vi "WPILib Camera Set Attributes From File.vi"(8 "error in":errorcluster, 10 "Config Path":path, 11 "CameraDevRef":T1) -> (0 "error out":errorcluster, 3 "CameraDevRef":T1)   [LabVIEW 2015]
uses:
  <vilib>/Rock Robotics/WPI/Camera/WPI_CameraDevRef.ctl
  <vilib>/userdefined/High Color/IMAQdx.ctl
  <vilib>/Utility/file.llb/Read Delimited Spreadsheet (string).vi
  <resource>/objmgr/imaqdx.rc
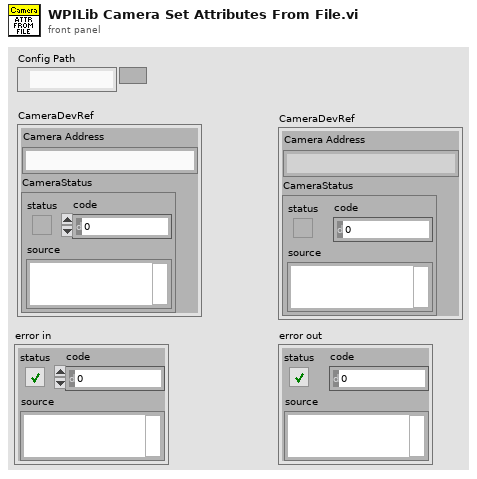
[diagram p1: front panel]
types:
  T1 = typedef "WPI_CameraDevRef.ctl" = cluster{"Camera Address":string, "CameraStatus":errorcluster}
  T2 = typedef "IMAQdx.ctl" = refnum<k21>
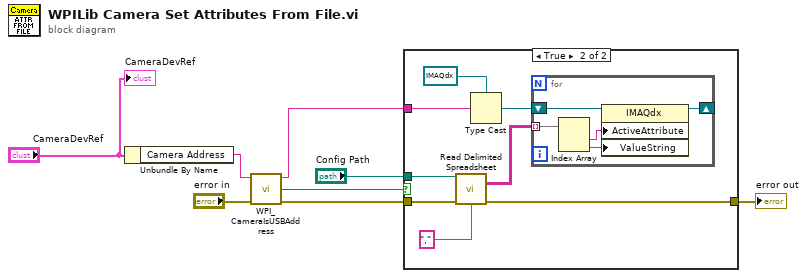
[diagram p0: block diagram]
diagram:
  n1 = Unbundle By Name("CameraDevRef") -> ("Camera Address"=w6:string)
  n2 = call <vilib>:"WPI_CameraIsUSBAddress.vi"("error in (no error)"="error in", "Camera Address In"=w6) -> ("error out"=w3:errorcluster, "USB?"=w1:bool, "Camera Address Out"=w7:string)  [unwired: 7 in]
  n3 = case shown="True" w1 {
    tunnel: "Config Path" -> [_ w17]
    tunnel: w7 -> [_ w16]
    tunnel: w3 -> [w9 w11]
    tunnel: [w9 w10] -> w2
    frame False {
    }
    frame True {
      n4 = call-poly <vilib>:"Read Delimited Spreadsheet.vi"("file path (dialog if empty)"=w17, "error in (no error)"=w11, "delimiter (\\t)"="," ("delimiter (\\t)")) -> ("all rows"=w12:string[][], "error out"=w10:errorcluster)  [unwired: 7 in, 4 out]
      n5 = Type Cast(type=T2 refnum ("Session In"), x=w16) -> (*(type *) &x=w15:T2)
      n6 = for {
        shift-right: [w21] -> _
        shift-left: w15 -> [w22]
        tunnel: w12 -> [w20] mode=indexing
        n7 = Index Array(array=w20) -> (element #1=w19:string, element #2=w18:string)  [unwired: 2 in]
        n8 = property class="IMAQdx"(reference=w22, "ActiveAttribute"=w19, "ValueString"=w18) -> (reference out=w21:T2)  [unwired: 1 in, 1 out]
      }
    }
  }
  "error out" <- w2
  "CameraDevRef" <- "CameraDevRef"
